vi "R5CleanUp.vi"(8 "error in (no error)":errorcluster) -> (0 "error out":errorcluster)   [LabVIEW 2016]
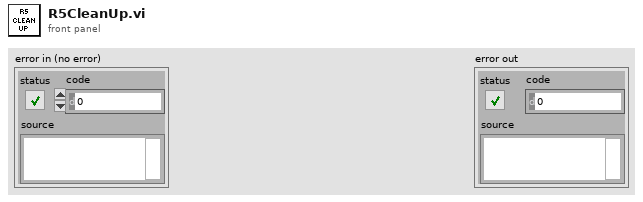
[diagram p1: front panel]
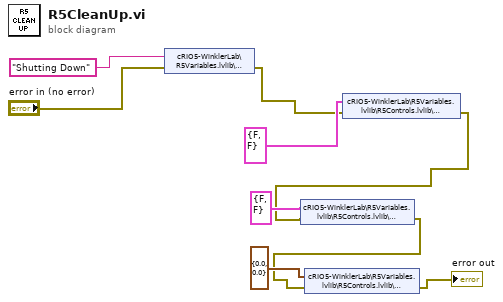
[diagram p0: block diagram]
diagram:
  n1 = shared-variable "cRIO5-WinklerLab\\R5Variables.lvlib\\R5Status"("Shutting Down" ("R1Status"), error in="error in (no error)") -> (error out=w1:errorcluster)
  n2 = shared-variable "cRIO5-WinklerLab\\R5Variables.lvlib\\R5Controls.lvlib\\R5SBRManual"(cluster{"Media Pump":bool, "Effluent Pump":bool} {"Media Pump"=FALSE, "Effluent Pump"=FALSE} ("R5SBRManual"), error in=w1) -> (error out=w7:errorcluster)
  n3 = shared-variable "cRIO5-WinklerLab\\R5Variables.lvlib\\R5Controls.lvlib\\R5pHManual"(cluster{"Acid Pump":bool, "Base Pump":bool} {"Acid Pump"=FALSE, "Base Pump"=FALSE} ("R1pHManual"), error in=w7) -> (error out=w5:errorcluster)
  n4 = shared-variable "cRIO5-WinklerLab\\R5Variables.lvlib\\R5Controls.lvlib\\R5DOManual"(cluster{"Air MFC":dbl, "N2 MFC":dbl} {"Air MFC"=0.0, "N2 MFC"=0.0} ("R1DOManual"), error in=w5) -> (error out=→"error out":errorcluster)
